vi "Find Center Angle in Radians.vi"(7 "output range (-pi to pi)":T1=enum."-pi to pi", 9 "right angle (rad)":dbl, 11 "left angle (rad)":dbl) -> (2 "center angle (rad)":dbl)   [LabVIEW 2017, in "NI_Robotics Utilities.lvlib"]
doc: "This VI is deprecated. Use <vi.lib>\\Analysis\\coordinate.llb\\Find Center Angle.vi instead."
uses:
  <vilib>/robotics/Utilities/NI_Robotics Utilities.lvlib
  <vilib>/robotics/Utilities/Angle Range_Radians.ctl
  <vilib>/robotics/Utilities/Rotate Angle in Radians (Scalar).vi
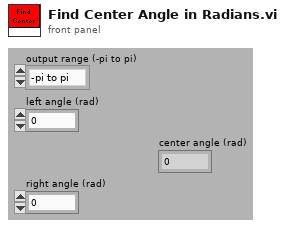
[diagram p1: front panel]
types:
  T1 = typedef "NI_Robotics Utilities.lvlib/Angle Range_Radians.ctl" = enum16{"none", "-pi to pi", "0 to 2*pi"}
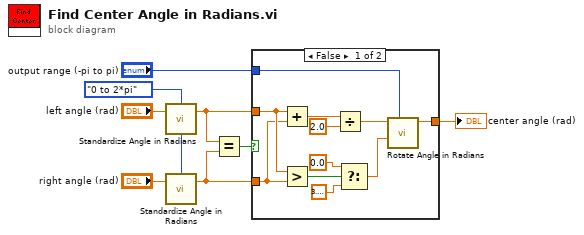
[diagram p0: block diagram]
diagram:
  w1 = Angle_Range_Radians."0 to 2*pi" ("range (-pi to pi)")
  n1 = call <vilib>:"Standardize Angle in Radians.vi"("angle in (rad)"="left angle (rad)", "range (-pi to pi)"=w1) -> ("angle out (rad)"=w5:dbl)  [unwired: 3 in]
  n2 = call <vilib>:"Standardize Angle in Radians.vi"("angle in (rad)"="right angle (rad)", "range (-pi to pi)"=w1) -> ("angle out (rad)"=w6:dbl)  [unwired: 3 in]
  n3 = Equal?(x=w5, y=w6) -> (x = y?=w4:bool)
  n4 = case shown="False" w4 {
    tunnel: [w15 w20] -> w3
    tunnel: w6 -> [w17 _]
    tunnel: w5 -> [w18 w20]
    tunnel: "output range (-pi to pi)" -> [w14 _]
    frame False {
      n5 = Add(x=w18, y=w17) -> (x+y=w19:dbl)
      n6 = Greater?(x=w18, y=w17) -> (0:w12:bool)
      n7 = Divide(x=w19, y=2.0) -> (x/y=w13:dbl)
      n8 = Select(t=0.0, s=w12, f=3.141592653589793) -> (s? t:f=w9:dbl)
      n9 = call-poly <vilib>:"Rotate Angle in Radians.vi"("output range (-pi to pi)"=w14, "ccw rotation (rad)"=w9, "angle in (rad)"=w13) -> ("angle out (rad)"=w15:dbl)  [unwired: 8 in]
    }
    frame True {
    }
  }
  "center angle (rad)" <- w3
